vi "UpdateCoordinateSys.vi"(8 "error in (no error)":errorcluster, 10 "CoordinatteEntry":T2={"ProcessSetting"=[], "Project Name"="Parttern", "AnalysisSetting"=[], "Coord?"=FALSE, "OriginPointInfo"={"Output Original"=FALSE, "Origin Name"="", "Angle"=0.0, "Mode"=0, "OriginPoint"={"X"=0.0, "Y"=0.0}}, "CaliperSetting"=[], "CoordIndex"=[]} {"CaliperSetting"."CaliperEntry"."CaliperType" items=["Distance", "Mid Point", "Perpendicular Projection", "Lines Intersection", "Angle from Horizontal", "Angle from Vertical", "Angle Defined by 3 Points", "Angle Defined by 4 Points", "Bissecting Line", "Mid Line", "Center of Mass", "Area", "Line Fit", "Circle Fit", "Ellipse Fit"]; "OriginPointInfo"."Mode" items=["Horizontal Motion", "Vertical Motion", "Horizontal and Vertical Motion", "Horizontal. Vertical and Angular Motion"]; "AnalysisSetting"."ROI"."Contours"."Type" items=["No Selection", "Point", "Line", "Rectangle", "Oval", "Polygon", "Freehand Region", "Annulus", "Unused2", "Unused3", "Broken Line", "Freehand Line", "Rotated Rectangle"]}) -> (0 "error out":errorcluster, 1 "Coordinate System Out":T1 {"Measurement System"."Axis Reference" items=["Direct", "Indirect"]; "Measurement System"."Angle (deg)" format="%.2f"; "Measurement System"."Origin"."Y" format="%.2f"; "Measurement System"."Origin"."X" format="%.2f"; "Reference System"."Axis Reference" items=["Direct", "Indirect"]; "Reference System"."Angle (deg)" format="%.2f"; "Reference System"."Origin"."Y" format="%.2f"; "Reference System"."Origin"."X" format="%.2f"})   [LabVIEW 2019]
uses:
  Control/CoordinatteEntry.ctl
  Process/Controls/Process_Setting.ctl
  Ctrl/VisionProcessName.ctl
  Control/CoordinateAnalysisSetting.ctl
  Control/CoordinateCaliperSetting.ctl
  Caliper/Controls/CaliperDataEntry.ctl
  Caliper/Controls/CaliperType.ctl
  Caliper/Controls/SelectionListEntry.ctl
  Caliper/Controls/SelectionListEntryPointType.ctl
  Caliper/Controls/CaliperResult.ctl
  Analysis/Controls/Parttern Match/Analysis_PatternMatch_ResultWithnumber.ctl
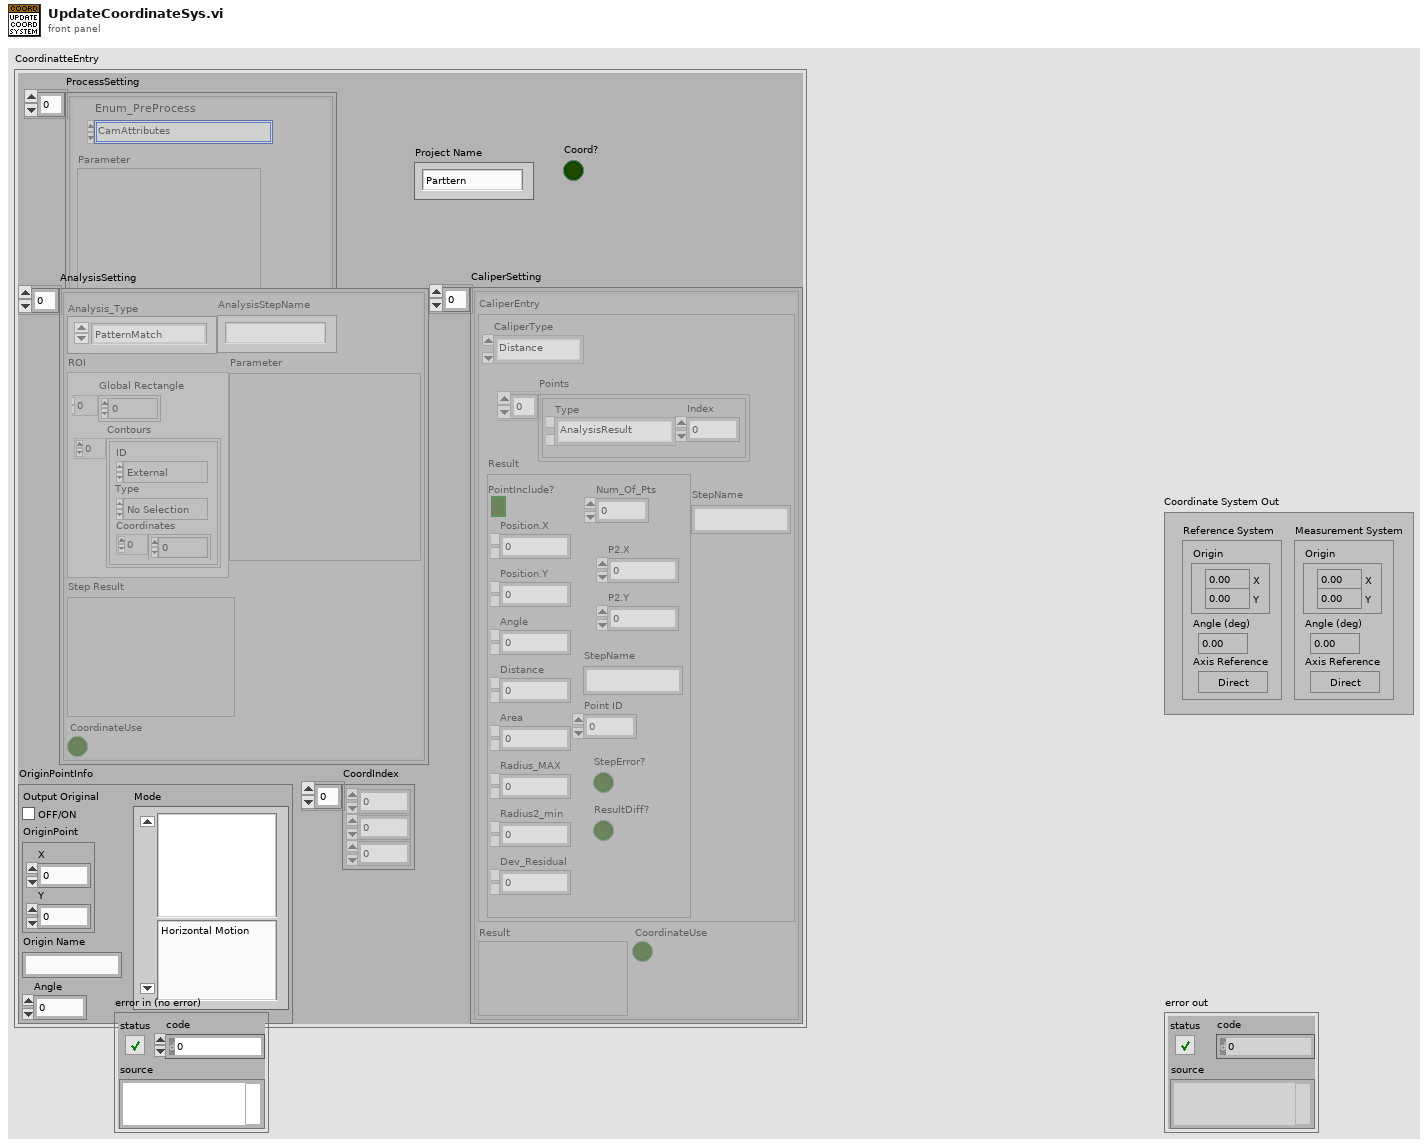
[diagram p1: front panel]
types:
  T1 = typedef "IMAQ Coordinate System" = cluster{"Reference System":cluster{"Origin":cluster{"X":sgl, "Y":sgl}, "Angle (deg)":sgl, "Axis Reference":u32}, "Measurement System":cluster{"Origin":cluster{"X":sgl, "Y":sgl}, "Angle (deg)":sgl, "Axis Reference":u32}}
  T2 = typedef "CoordinatteEntry.ctl" = cluster{"ProcessSetting":T3[], "Project Name":string, "AnalysisSetting":T5[], "Coord?":bool, "OriginPointInfo":cluster{"Output Original":bool, "Origin Name":string, "Angle":dbl, "Mode":u16, "OriginPoint":cluster{"X":dbl, "Y":dbl}}, "CaliperSetting":T7[], "CoordIndex":i32[]}
  T3 = typedef "Process_Setting.ctl" = cluster{"Enum_PreProcess":T4, "Parameter":string}
  T4 = typedef "VisionProcessName.ctl" = enum16{"*CamParameter*", "CamAttributes", "*Preprocess*", "CG_Brightness", "C_Plane Extraction", "C_Threshold", "G_Lookup Table", "G_Threshold"}
  T5 = typedef "CoordinateAnalysisSetting.ctl" = cluster{"Analysis_Type":enum16{"PatternMatch", "Straight Edge"}, "ROI ":T6, "Parameter":variant, "Step Result":variant, "AnalysisStepName":string, "CoordinateUse":bool}
  T6 = typedef "ROI Descriptor" = cluster{"Global Rectangle":i32[], "Contours":cluster{"ID":enum32{"External", "Internal"}, "Type":u32, "Coordinates":i32[]}[]}
  T7 = typedef "CoordinateCaliperSetting.ctl" = cluster{"Result":variant, "CoordinateUse":bool, "CaliperEntry":T8}
  T8 = typedef "CaliperDataEntry.ctl" = cluster{"CaliperType":T9, "Points":T10[], "Result":T12, "StepName":string}
  T9 = typedef "CaliperType.ctl" = u32
  T10 = typedef "SelectionListEntry.ctl" = cluster{"Type":T11, "Index":i32}
  T11 = typedef "SelectionListEntryPointType.ctl" = enum16{"AnalysisResult", "CaliperResult"}
  T12 = typedef "CaliperResult.ctl" = cluster{"PointInclude?":bool, "Num_Of_Pts":u8, "Position.X":dbl, "Position.Y":dbl, "Angle":dbl, "Distance":dbl, "Area":dbl, "Radius_MAX":dbl, "Radius2_min":dbl, "Dev_Residual":dbl, "P2.X":dbl, "P2.Y":dbl, "StepName":string, "Point ID":u8, "StepError?":bool, "ResultDiff?":bool}
  T13 = cluster{"Output Original":bool, "Origin Name":string, "Angle":dbl, "Mode":u16, "OriginPoint":cluster{"X":dbl, "Y":dbl}}
  T14 = typedef "Analysis_PatternMatch_ResultWithnumber.ctl" = cluster{"numbers":i32, "results":cluster{"ROI Descriptor out":T6, "Point":T15, "Angle":sgl, "Score":sgl, "Real World Coordinates":cluster{"X":sgl, "Y":sgl}, "Rectangle":T16}[]}
  T15 = typedef "IMAQ Point" = cluster{"X":sgl, "Y":sgl}
  T16 = typedef "IMAQ Rectangle" = cluster{"Left":i32, "Top":i32, "Right":i32, "Bottom":i32, "Rotation":dbl}
  T17 = cluster{"Point1 (Pixels)":cluster{"X":sgl, "Y":sgl}, "Point2 (Pixels)":cluster{"X":sgl, "Y":sgl}, "Point1 (Real-World)":cluster{"X":sgl, "Y":sgl}, "Point2 (Real-World)":cluster{"X":sgl, "Y":sgl}, "Angle (Pixel)":dbl, "Angle (Real-World)":dbl, "Score":dbl, "Straightness":dbl, "Average SNR (db)":dbl, "Calibration Valid":bool}[]
  T18 = cluster{"ROI Descriptor out":T6, "Point":T15, "Angle":sgl, "Score":sgl, "Real World Coordinates":cluster{"X":sgl, "Y":sgl}, "Rectangle":T16}[]
  T19 = cluster{"ROI Descriptor out":T6, "Point":T15, "Angle":sgl, "Score":sgl, "Real World Coordinates":cluster{"X":sgl, "Y":sgl}, "Rectangle":T16}
  T20 = cluster{"Point1 (Pixels)":cluster{"X":sgl, "Y":sgl}, "Point2 (Pixels)":cluster{"X":sgl, "Y":sgl}, "Point1 (Real-World)":cluster{"X":sgl, "Y":sgl}, "Point2 (Real-World)":cluster{"X":sgl, "Y":sgl}, "Angle (Pixel)":dbl, "Angle (Real-World)":dbl, "Score":dbl, "Straightness":dbl, "Average SNR (db)":dbl, "Calibration Valid":bool}
  T21 = cluster{"OriginPoint":cluster{"X":dbl, "Y":dbl}, "Angle":dbl, "Axis Reference":u32}
  T22 = cluster{cluster{"Angle":dbl, "Angle":dbl}, "Angle":dbl, "Axis Reference":u32}
  T23 = cluster{cluster{"OriginPoint":cluster{"X":dbl, "Y":dbl}, "Angle":dbl, "Axis Reference":u32}, cluster{cluster{"Angle":dbl, "Angle":dbl}, "Angle":dbl, "Axis Reference":u32}}
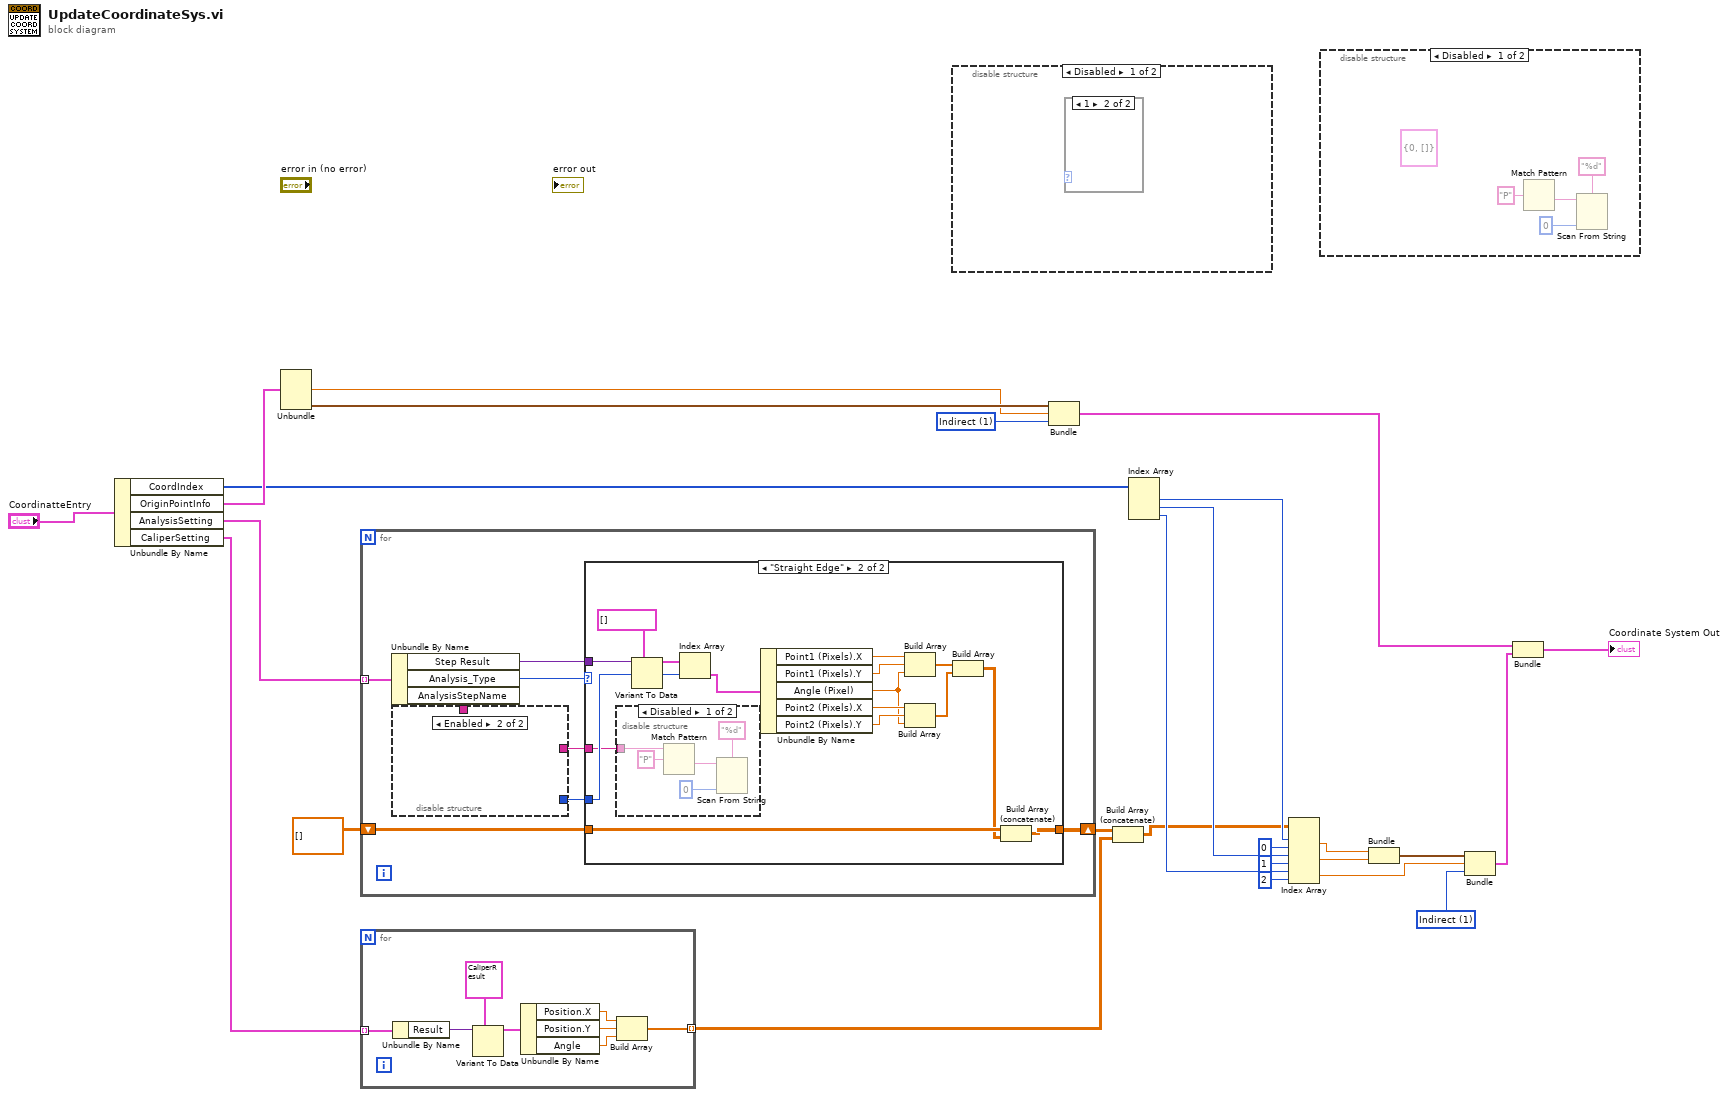
[diagram p0: block diagram]
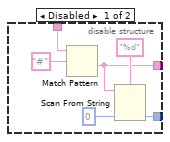
[diagram p4: hidden frame]
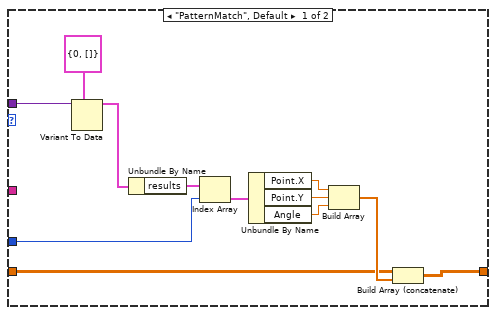
[diagram p5: hidden frame]
diagram:
  w20 = u32 1 items=["Direct", "Indirect"] ("Axis Reference")
  w22 = u32 1 items=["Direct", "Indirect"] ("Axis Reference")
  n1 = Unbundle By Name("CoordinatteEntry") -> ("CoordIndex"=w14:i32[], "OriginPointInfo"=w25:T13, "AnalysisSetting"=w17:T5[], "CaliperSetting"=w18:T7[])
  n2 = Unbundle(w25) -> ("Angle"=w23:dbl, "OriginPoint"=w24:cluster{"X":dbl, "Y":dbl})  [unwired: 3 out]
  n3 = for {
    tunnel: w17 -> [w34] mode=indexing
    shift-right: [w29] -> w15
    shift-left: dbl[][] [] -> [w28]
    n4 = Unbundle By Name(w34) -> ("Step Result"=w30:variant, "Analysis_Type"=w33:enum16{"PatternMatch", "Straight Edge"}, "AnalysisStepName"=w27:string)
    n5 = disable-structure shown="Enabled" {
      disable-tunnel: [w37 _] -> w32
      disable-tunnel: [w36 _] -> w31
      disable-tunnel: w27 -> [w35 _]
      frame Disabled {
        n6 = Match Pattern(string=w35, regular expression="#") -> (after substring=w36:string)  [unwired: 1 in, 3 out]
        n7 = Scan From String(format string="%d", input string=w36, default 1=0) -> (output 1=w37:i32)  [unwired: 2 in, 3 out]
      }
      frame Enabled {
      }
    }
    n8 = case shown="\"Straight Edge\"" w33 {
      tunnel: w30 -> [w52 w68]
      tunnel: w32 -> [w51 w65]
      tunnel: [w42 w53] -> w29
      tunnel: w31 -> [_ w63]
      tunnel: w28 -> [w41 w55]
      frame "PatternMatch", Default {
        n9 = Variant To Data(type=T14 {"numbers"=0, "results"=[]} ("PatternMatchResult"), Variant=w52) -> (data=w46:T14)  [unwired: 1 in, 1 out]
        n10 = Unbundle By Name(w46) -> ("results"=w45:T18)
        n11 = Index Array(array=w45, index=w51) -> (element=w50:T19)
        n12 = Unbundle By Name(w50) -> ("Point.X"=w49:sgl, "Point.Y"=w48:sgl, "Angle"=w44:sgl)
        n13 = Build Array(w49, w48, w44) -> (w43:sgl[])
        n14 = Build Array (concatenate)(w41, w43) -> (w42:dbl[][])
      }
      frame "Straight Edge" {
        n15 = disable-structure shown="Disabled" {
          disable-tunnel: w63 -> [w73 _]
          frame Disabled {
            n16 = Match Pattern(string=w73, regular expression="P") -> (after substring=w71:string)  [unwired: 1 in, 3 out]
            n17 = Scan From String(format string="%d", input string=w71, default 1=0) -> ()  [unwired: 3 in, 3 out]
          }
          frame Enabled {
          }
        }
        n18 = Variant To Data(type=T17 [], Variant=w68) -> (data=w66:T17)  [unwired: 1 in, 1 out]
        n19 = Index Array(array=w66, index=w65) -> (element=w64:T20)
        n20 = Unbundle By Name(w64) -> ("Point1 (Pixels).X"=w62:sgl, "Point1 (Pixels).Y"=w61:sgl, "Angle (Pixel)"=w58:dbl, "Point2 (Pixels).X"=w60:sgl, "Point2 (Pixels).Y"=w59:sgl)
        n21 = Build Array(w62, w61, w58) -> (w57:dbl[])
        n22 = Build Array(w60, w59, w58) -> (w56:dbl[])
        n23 = Build Array(w57, w56) -> (w54:dbl[][])
        n24 = Build Array (concatenate)(w55, w54) -> (w53:dbl[][])
      }
    }
  }
  n25 = for {
    tunnel: w18 -> [w81] mode=indexing
    tunnel: [w74] -> w1 mode=indexing
    n26 = Unbundle By Name(w81) -> ("Result"=w80:variant)
    n27 = Variant To Data(type=T12 {"PointInclude?"=FALSE, "Num_Of_Pts"=0, "Position.X"=0.0, "Position.Y"=0.0, "Angle"=0.0, "Distance"=0.0, "Area"=0.0, "Radius_MAX"=0.0, "Radius2_min"=0.0, "Dev_Residual"=0.0, "P2.X"=0.0, "P2.Y"=0.0, "StepName"="", "Point ID"=0, "StepError?"=FALSE, "ResultDiff?"=FALSE} ("Result"), Variant=w80) -> (data=w79:T12)  [unwired: 1 in, 1 out]
    n28 = Unbundle By Name(w79) -> ("Position.X"=w75:dbl, "Position.Y"=w76:dbl, "Angle"=w77:dbl)
    n29 = Build Array(w75, w76, w77) -> (w74:dbl[])
  }
  n30 = disable-structure shown="Disabled" {
    frame Disabled {
      n31 = case shown="1" {
        selector: _ -> [_ _]
        frame 0, Default {
        }
        frame 1 {
        }
      }
    }
    frame Enabled {
    }
  }
  n32 = Bundle("OriginPoint"=w24, "Angle"=w23, "Axis Reference"=w22) -> (w21:T21)  [unwired: 1 in]
  n33 = Build Array (concatenate)(w15, w1) -> (w2:dbl[][])
  n34 = Index Array(array=w14) -> (element #1=w12:i32, element #2=w11:i32, element #3=w13:i32)  [unwired: 3 in]
  n35 = Index Array(array=w2, index (row) #1=w12, index (col) #1=0 ("disabled index (col)"), index (row) #2=w11, index (col) #2=1 ("disabled index (col)"), index (row) #3=w13, index (col) #3=2 ("disabled index (col)")) -> (element #1=w7:dbl, element #2=w6:dbl, element #3=w4:dbl)
  n36 = disable-structure shown="Disabled" {
    frame Disabled {
      (unwired) T14 {"numbers"=0, "results"=[]} ("PatternMatchResult")
      n37 = Match Pattern(regular expression="P") -> (after substring=w83:string)  [unwired: 2 in, 3 out]
      n38 = Scan From String(format string="%d", input string=w83, default 1=0) -> ()  [unwired: 3 in, 3 out]
    }
    frame Enabled {
    }
  }
  n39 = Bundle("Angle"=w7, "Angle"=w6) -> (w5:cluster{"Angle":dbl, "Angle":dbl})  [unwired: 1 in]
  n40 = Bundle(w5, "Angle"=w4, "Axis Reference"=w20) -> (w19:T22)  [unwired: 1 in]
  n41 = Bundle(w21, w19) -> (→"Coordinate System Out":T23)  [unwired: 1 in]
